vi "Main_EvaluateRotNoise.vi"() -> ()   [LabVIEW 2020]
panel:
  in  "Tab Control":T1(tab)
  in  "Num of Sim":i32=100
  out "XYグラフ":T2(graph)
  in  "Select Mol Posi":u16(ring)=4 items=["3-motors", "5-motors", "7-motors", "9-motors", "13-motors", "13-motors-sparse", "19-motors", ""]
  in  "SD":dbl=0.11000000000000001
  in  "Tau_On":i32=40
  in  "Tau_Off":i32=10
  in  "Sim time":i32=25000
  in  "Asymmetry (X, Y)":dbl[](array[numeric])=[0.12000000000000001, 0.58]
  out "Counter":i32
  in  "Torque":bool=TRUE
  in  "Torque (deg)":dbl=-4.0
  in  "停止":bool
  in  "Rot_Noise for Cargo":bool=TRUE
  in  "Width of Rot_Noise (deg)":dbl=8.0 format="%#_13g"
  in  "SaveData":bool
  out "Counter":i32
  in  "Ini_Posi (19 mol)":dbl[][](array[numeric])=[[0.0, 0.0], [12.0, 0.0], [-12.0, 0.0], [9.0, 3.0], [-9.0, 3.0], [9.0, -3.0], [-9.0, -3.0], [6.0, 0.0], [-6.0, 0.0], [0.0, 6.0], [0.0, -6.0], [6.0, 6.0], [6.0, -6.0], [-6.0, 6.0], [-6.0, -6.0], [3.0, 3.0], [3.0, -3.0], [-3.0, 3.0], [-3.0, -3.0]]
  in  "Ini_Posi (3 mol)":dbl[][](array[numeric])=[[0.0, 0.0], [6.0, 0.0], [-6.0, 0.0]]
  in  "Ini_Posi (5 mol)":dbl[][](array[numeric])=[[0.0, 0.0], [6.0, 0.0], [-6.0, 0.0], [0.0, 6.0], [0.0, -6.0]]
  in  "Ini_Posi (9 mol)":dbl[][](array[numeric])=[[0.0, 0.0], [6.0, 0.0], [-6.0, 0.0], [0.0, 6.0], [0.0, -6.0], [6.0, 6.0], [6.0, -6.0], [-6.0, 6.0], [-6.0, -6.0]]
  in  "Ini_Posi (13 mol)":dbl[][](array[numeric])=[[0.0, 0.0], [6.0, 0.0], [-6.0, 0.0], [0.0, 6.0], [0.0, -6.0], [6.0, 6.0], [6.0, -6.0], [-6.0, 6.0], [-6.0, -6.0], [3.0, 3.0], [3.0, -3.0], [-3.0, 3.0], [-3.0, -3.0]]
  in  "Ini_Posi (13 mol#2)":dbl[][](array[numeric])=[[0.0, 0.0], [17.0, 0.0], [-17.0, 0.0], [17.0, 9.0], [-17.0, 9.0], [17.0, -9.0], [-17.0, -9.0], [9.0, 0.0], [-9.0, 0.0], [9.0, 9.0], [9.0, -9.0], [-9.0, 9.0], [-9.0, -9.0]]
  in  "Ini_Posi (7 mol)":dbl[][](array[numeric])=[[0.0, 0.0], [5.0, 3.0], [-5.0, 3.0], [5.0, -3.0], [-5.0, -3.0], [0.0, 6.0], [0.0, -6.0]]
  out "Y":dbl[](graph)
  out "XY-trace":cluster{"Position":dbl[], "Position":dbl[]}[](graph)
  out "Angle":dbl[](graph)
  out "Num of On-Particles":dbl[](graph)
  out "Cross Corr":dbl[](graph)
  out "Corr_Coef_Pearson":T3
  out "Averaged CrossCorr":dbl[](graph)
  out "Graph_for_Coef":dbl[](graph)
  # "If you want to save data, press the button \nbefore you start simulations.\nSaved data contain time, Y-displacement, \nand angle."
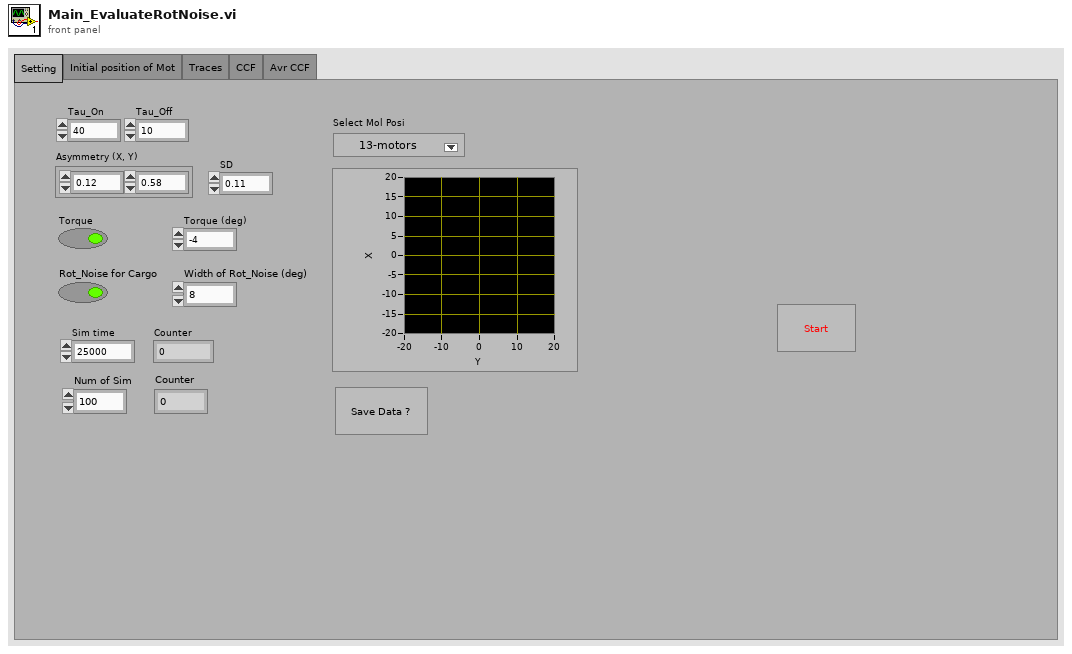
[diagram p1: front panel]
types:
  T1 = enum32{"Setting", "Initial position of Mot", "Traces", "CCF", "Avr CCF"}
  T2 = cluster{"Ini_Anchor_Posi (17 mol)":dbl[], "Ini_Anchor_Posi (17 mol)":dbl[]}
  T3 = cluster{"correlation coefficient r":dbl, "r^2":dbl}
  T4 = cluster{"Ini_Posi (19 mol) ":dbl[], "Ini_Posi (19 mol) ":dbl[]}
  T5 = cluster{"Center Position":dbl[], "Center Angle":dbl}
  T6 = cluster{"On/Off":bool, "Position":dbl[], "Dwell Count":i32}[]
  T7 = enum16{"open", "replace", "create", "open or create", "replace or create", "replace or create with confirmation"}
  T8 = cluster{"On/Off":bool, "Position":dbl[], "Next Dwell":i32}[]
  T9 = cluster{"On/Off":bool, "Position":dbl[], "Next Dwell":i32}
  T10 = cluster{"Center Position":dbl[], "Center Position":dbl[]}
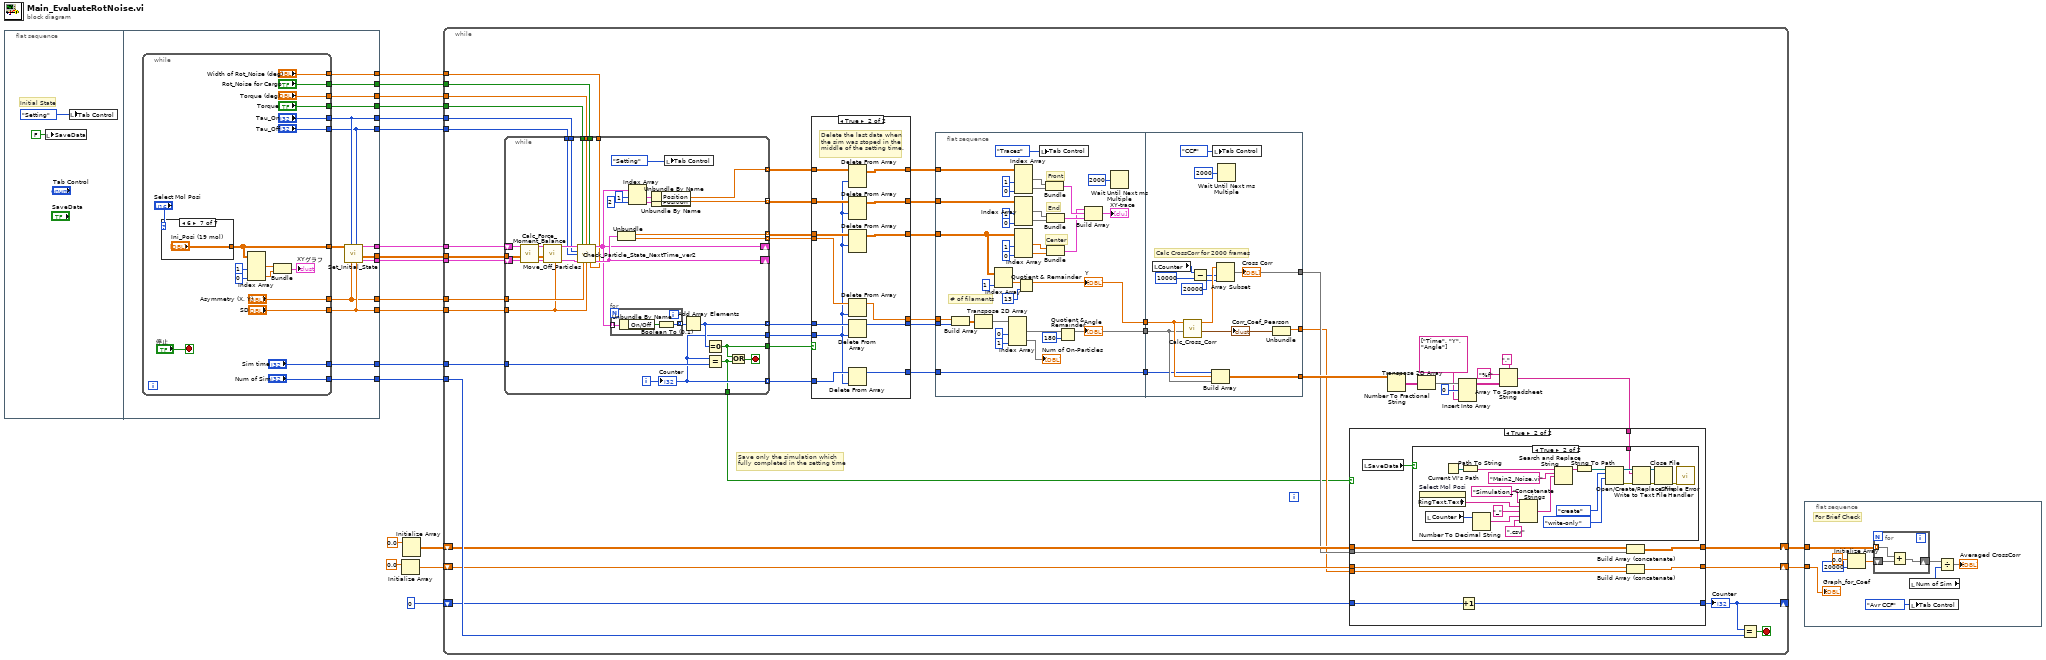
[diagram p0: block diagram]
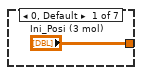
[diagram p5: hidden frame]
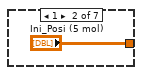
[diagram p6: hidden frame]
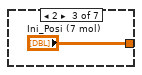
[diagram p7: hidden frame]
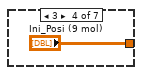
[diagram p8: hidden frame]
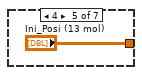
[diagram p9: hidden frame]
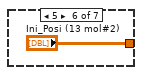
[diagram p10: hidden frame]
diagram:
  n1 = flat-sequence {
    tunnel: [w36] -> w20
    tunnel: [w35] -> w19
    tunnel: [w34] -> w18
    tunnel: [w31] -> w14
    tunnel: [w33] -> w17
    tunnel: [w32] -> w16
    tunnel: [w30] -> w15
    tunnel: [w29] -> w13
    tunnel: [w28] -> w12
    tunnel: [w26] -> w11
    tunnel: [w25] -> w10
    tunnel: [w24] -> w9
    tunnel: [w23] -> w8
    frame #0 {
      # "Initial State"
      n2 = local write "SaveData"(FALSE ("SaveData")) -> ()
      n3 = local write "Tab Control"(T1."Setting" ("Tab Control")) -> ()
    }
    frame #1 {
      n4 = while {
        tunnel: ["Tau_On"] -> w33
        tunnel: ["Tau_Off"] -> w32
        tunnel: ["SD"] -> w31
        tunnel: ["Asymmetry (X, Y)"] -> w30
        tunnel: ["Torque"] -> w29
        tunnel: ["Torque (deg)"] -> w28
        tunnel: [w48] -> w27
        tunnel: ["Rot_Noise for Cargo"] -> w26
        tunnel: ["Width of Rot_Noise (deg)"] -> w25
        tunnel: ["Sim time"] -> w24
        tunnel: ["Num of Sim"] -> w23
        stop <- "停止" stop-if-true
        n5 = case shown="6" "Select Mol Posi" {
          tunnel: ["Ini_Posi (3 mol)" "Ini_Posi (5 mol)" "Ini_Posi (7 mol)" "Ini_Posi (9 mol)" "Ini_Posi (13 mol)" "Ini_Posi (13 mol#2)" "Ini_Posi (19 mol)"] -> w48
          frame 0, Default {
          }
          frame 1 {
          }
          frame 2 {
          }
          frame 3 {
          }
          frame 4 {
          }
          frame 5 {
          }
          frame 6 {
          }
        }
        n6 = Index Array(array=w48, index (col) #1=1 ("無効な指標 (列)"), index (col) #2=0 ("指標 (列)")) -> (element #1=w43:dbl[], element #2=w42:dbl[])  [unwired: 2 in]
        n7 = Bundle("Ini_Posi (19 mol)"=w43, "Ini_Posi (19 mol)"=w42) -> (→"XYグラフ":T4)  [unwired: 1 in]
      }
      n8 = call "Set_Initial_State.vi"("SD"=w31, "Tau_Off"=w32, "Asymmetry (X, Y)"=w30, "Tau_On"=w33, "Ini_Anchor_Posi"=w27) -> ("Center State at T"=w34:T5, "Ini_Anchor_Posi"=w35:dbl[][], "On_Particle State"=w36:T6)  [unwired: 4 in]
    }
  }
  n9 = Initialize Array(0.0 ("要素")) -> (w6:dbl[])  [unwired: 1 in]
  n10 = Initialize Array(0.0 ("要素")) -> (w4:dbl[][])  [unwired: 2 in]
  n11 = while {
    tunnel: w20 -> [w110]
    tunnel: w19 -> [w109]
    tunnel: w18 -> [w108]
    tunnel: w17 -> [w107]
    tunnel: w16 -> [w106]
    tunnel: w15 -> [w105]
    tunnel: w14 -> [w104]
    tunnel: w13 -> [w103]
    tunnel: w12 -> [w102]
    tunnel: w11 -> [w96]
    tunnel: w10 -> [w95]
    tunnel: w9 -> [w94]
    tunnel: w8 -> [w92]
    shift-right: [w67] -> w2
    shift-left: w6 -> [w68]
    shift-right: [w70] -> w3
    shift-left: w4 -> [w69]
    shift-right: [w63] -> _
    shift-left: 0 -> [w64]
    stop <- w93 stop-if-true
    # "Save only the simulation which \nfully completed in the setting time"
    n12 = while {
      tunnel: w109 -> [w195]
      shift-right: [w186] -> _
      shift-left: w108 -> [w193]
      shift-right: [w179] -> _
      shift-left: w110 -> [w194]
      tunnel: w107 -> [w185]
      tunnel: w106 -> [w184]
      tunnel: w105 -> [w181]
      tunnel: w104 -> [w180]
      tunnel: w103 -> [w182]
      tunnel: w102 -> [w183]
      tunnel: w94 -> [w166]
      tunnel: [w174] -> w89
      tunnel: [w165] -> w88
      tunnel: w96 -> [w173]
      tunnel: w95 -> [w172]
      tunnel: [w171] -> w87 mode=indexing
      tunnel: [w170] -> w86 mode=indexing
      tunnel: [w169] -> w85 mode=indexing
      tunnel: [w168] -> w84 mode=indexing
      tunnel: [w167] -> w83 mode=indexing
      tunnel: [w165] -> w82 mode=indexing
      tunnel: [w164] -> w62
      i -> [w165]
      stop <- w175 stop-if-true
      n13 = call "Calc_Force_Moment_Balance.vi"("Center State at T"=w193, "Ini_Anchor_Posi"=w195, "On_Particle State"=w194) -> ("New Center State at T"=w188:T5, "Ini_Anchor_Posi"=w189:dbl[][], "On_Particle State"=w196:T6)  [unwired: 6 in]
      n14 = call "Move_Off_Particles.vi"("SD"=w180, "Center State at T"=w188, "Ini_Anchor_Posi"=w189, "Particle Posi at T"=w196) -> ("Center State at T"=w187:T5, "New Particle Posi at T"=w190:T8)  [unwired: 6 in]
      n15 = call "Check_Particle_State_NextTime_ver2.vi"("Particle State at T"=w190, "Torque?"=w182, "Torque"=w183, "Rot diffusion\nfor Cargo?"=w173, "Tau_On"=w185, "Tau_Off"=w184, "Center State at T"=w187, "Asymmetry (X, Y)"=w181, "SD"=w180, "Rot diffusion\nfor Cargo"=w172) -> ("Particle State at T+1"=w179:T8, "New Center State at T"=w186:T5)  [unwired: 4 in]
      n16 = for {
        tunnel: w179 -> [w199] mode=indexing
        tunnel: [w197] -> w178 mode=indexing
        n17 = Unbundle By Name(w199) -> ("On/Off"=w198:bool)
        n18 = Boolean To (0,1)(Boolean=w198) -> (0, 1=w197:i16)
      }
      n19 = Unbundle(w186) -> ("Center Position"=w169:dbl[], "Center Angle"=w168:dbl)
      n20 = Index Array(array=w179, index #1=1 ("index"), index #2=2 ("index")) -> (element #1=w192:T9, element #2=w191:T9)
      n21 = Unbundle By Name(w192) -> ("Position"=w171:dbl[])
      n22 = Unbundle By Name(w191) -> ("Position"=w170:dbl[])
      n23 = local write "Tab Control"(T1."Setting" ("Tab Control")) -> ()
      n24 = Add Array Elements(numeric array=w178) -> (sum=w167:i16)
      n25 = Equal To 0?(x=w167) -> (x = 0?=w174:bool)
      n26 = Equal?(x=w165, y=w166) -> (x = y?=w164:bool)
      n27 = Or(x=w174, y=w164) -> (x .or. y?=w175:bool)
      "Counter" <- w165
    }
    n28 = case shown="TRUE" w89 {
      tunnel: w87 -> [w149 w162]
      tunnel: w86 -> [w148 w161]
      tunnel: w88 -> [_ w151]
      tunnel: w85 -> [w147 w160]
      tunnel: w84 -> [w146 w159]
      tunnel: w83 -> [w145 w158]
      tunnel: [w145 w157] -> w101
      tunnel: [w146 w156] -> w100
      tunnel: [w147 w155] -> w99
      tunnel: [w148 w154] -> w98
      tunnel: [w149 w153] -> w97
      tunnel: w82 -> [w144 w152]
      tunnel: [w144 w150] -> w81
      frame False {
      }
      frame True {
        # "Delete the last data when \nthe sim was stoped in the\nmiddle of the setting time."
        n29 = Delete From Array(array=w162, index (row)=w151) -> (array with subset deleted=w153:dbl[][])  [unwired: 2 in, 1 out]
        n30 = Delete From Array(array=w161, index (row)=w151) -> (array with subset deleted=w154:dbl[][])  [unwired: 2 in, 1 out]
        n31 = Delete From Array(array=w160, index (row)=w151) -> (array with subset deleted=w155:dbl[][])  [unwired: 2 in, 1 out]
        n32 = Delete From Array(array=w159, index=w151) -> (array with subset deleted=w156:dbl[])  [unwired: 1 in, 1 out]
        n33 = Delete From Array(array=w158, index=w151) -> (array with subset deleted=w157:i16[])  [unwired: 1 in, 1 out]
        n34 = Delete From Array(array=w152, index=w151) -> (array with subset deleted=w150:i32[])  [unwired: 1 in, 1 out]
      }
    }
    n35 = flat-sequence {
      tunnel: w101 -> [w235]
      tunnel: w100 -> [w234]
      tunnel: w99 -> [w206]
      tunnel: w98 -> [w207]
      tunnel: w97 -> [w208]
      tunnel: [w204] -> w91
      tunnel: [w203] -> w90
      tunnel: w81 -> [w202]
      tunnel: [w202] -> w80
      tunnel: [w244] -> w66
      tunnel: w91 -> [w239]
      tunnel: w90 -> [w240]
      tunnel: [w241] -> w65
      tunnel: [w238] -> w79
      tunnel: w80 -> [w237]
      frame #0 {
        # "End"
        # "Front"
        # "Center"
        # "# of filaments"
        n36 = Build Array(w234, w235) -> (w233:dbl[][])
        n37 = Transpose 2D Array(2D array=w233) -> (transposed array=w205:dbl[][])
        n38 = Index Array(array=w206, index (col)=1 ("disabled index (col)")) -> (element=w226:dbl[])  [unwired: 1 in]
        n39 = Index Array(array=w205, index (col) #1=0 ("disabled index (col)"), index (col) #2=1 ("index (col)")) -> (element #1=w228:dbl[], element #2=→"Num of On-Particles":dbl[])  [unwired: 2 in]
        n40 = Index Array(array=w208, index (col) #1=1 ("disabled index (col)"), index (col) #2=0 ("index (col)")) -> (element #1=w212:dbl[], element #2=w221:dbl[])  [unwired: 2 in]
        n41 = Index Array(array=w207, index (col) #1=1 ("disabled index (col)"), index (col) #2=0 ("index (col)")) -> (element #1=w213:dbl[], element #2=w220:dbl[])  [unwired: 2 in]
        n42 = Index Array(array=w206, index (col) #1=1 ("disabled index (col)"), index (col) #2=0 ("index (col)")) -> (element #1=w211:dbl[], element #2=w215:dbl[])  [unwired: 2 in]
        n43 = Quotient & Remainder(x=w226, y=13) -> (x-y*floor(x/y)=w203:dbl[])  [unwired: 1 out]
        "Y" <- w203
        n44 = local write "Tab Control"(T1."Traces" ("Tab Control")) -> ()
        n45 = Bundle("Position"=w212, "Position"=w221) -> (w219:cluster{"Position":dbl[], "Position":dbl[]})  [unwired: 1 in]
        n46 = Bundle("Position"=w213, "Position"=w220) -> (w218:cluster{"Position":dbl[], "Position":dbl[]})  [unwired: 1 in]
        n47 = Bundle("Center Position"=w211, "Center Position"=w215) -> (w214:T10)  [unwired: 1 in]
        n48 = Quotient & Remainder(x=w228, y=180) -> (x-y*floor(x/y)=w204:dbl[])  [unwired: 1 out]
        "Angle" <- w204
        n49 = Build Array(w214, w219, w218) -> (→"XY-trace":cluster{"Position":dbl[], "Position":dbl[]}[])
        n50 = Wait Until Next ms Multiple(millisecond multiple=u32 2000 ("ミリ秒倍数")) -> ()  [unwired: 1 out]
      }
      frame #1 {
        # "Calc CrossCorr for 2000 frames"
        n51 = local read "Counter"() -> (w243:i32)
        n52 = call "Calc_Cross_Corr.vi"("Y"=w239, "X"=w240) -> ("Corr_Coef_Pearson"=w242:T3, "Cross"=w248:dbl[])  [unwired: 7 in, 1 out]
        "Corr_Coef_Pearson" <- w242
        n53 = Subtract(x=w243, y=10000) -> (x-y=w245:i32)
        n54 = Build Array(w237, w240, w239) -> (w238:dbl[][])
        n55 = local write "Tab Control"(T1."CCF" ("Tab Control")) -> ()
        n56 = Array Subset(array=w248, index=w245, length=20000 ("長さ")) -> (w244:dbl[])
        "Cross Corr" <- w244
        n57 = Wait Until Next ms Multiple(millisecond multiple=u32 2000 ("ミリ秒倍数")) -> ()  [unwired: 1 out]
        n58 = Unbundle(w242) -> ("correlation coefficient r"=w241:dbl)  [unwired: 1 out]
      }
    }
    n59 = Number To Fractional String(number=w79) -> (F-format string=w75:string[][])  [unwired: 3 in]
    n60 = Transpose 2D Array(2D array=w75) -> (transposed array=w78:string[][])
    n61 = Insert Into Array(array=w78, index (row)=0 ("指標 (行)"), new element=string[] ["Time", "Y", "Angle"]) -> (w73:string[][])  [unwired: 1 in]
    n62 = Array To Spreadsheet String(delimiter (Tab)=",", array=w73, 3:"%f" ("format string")) -> (spreadsheet string=w72:string)
    n63 = case shown="TRUE" w62 {
      tunnel: w72 -> [_ w123]
      tunnel: [w113 w121] -> w70
      tunnel: w69 -> [w113 w122]
      tunnel: [w112 w118] -> w67
      tunnel: w68 -> [w112 w119]
      tunnel: w66 -> [_ w120]
      tunnel: w65 -> [_ w117]
      tunnel: [w111 w116] -> w63
      tunnel: w64 -> [w111 w115]
      frame False {
      }
      frame True {
        n64 = local read "SaveData"() -> (w114:bool)
        n65 = case shown="TRUE" w114 {
          tunnel: w123 -> [_ w128]
          frame False {
          }
          frame True {
            n66 = property on="Select Mol Posi" class="Ring (指定)"() -> ("RingText.Text"=w129:string)  [unwired: 2 in, 2 out]
            n67 = local read "Counter"() -> (w127:i32)
            n68 = Current VI's Path() -> (path=w135:path)
            n69 = Path To String(path=w135) -> (string=w134:string)
            n70 = Number To Decimal String(number=w127) -> (decimal integer string=w125:string)  [unwired: 1 in]
            n71 = Concatenate Strings("Simulation_" ("文字列"), w129, "_" ("文字列"), w125, ".csv" ("string")) -> (w132:string)
            n72 = Search and Replace String(input string=w134, search string="Main2_Noise.vi", replace string=w132) -> (result string=w131:string)  [unwired: 5 in, 3 out]
            n73 = String To Path(string=w131) -> (path=w136:path)
            n74 = Open/Create/Replace File(file path (use dialog)=w136, operation (0:open)=T7."create", access (0:read/write)=enum16{"read/write", "read-only", "write-only"}."write-only") -> (refnum out=w139:refnum<file>, error out=w140:errorcluster)  [unwired: 1 in, 3 out]
            n75 = Write to Text File(file (use dialog)=w139, text=w128, error in=w140) -> (refnum out=w142:refnum<file>, error out=w143:errorcluster)  [unwired: 1 in, 1 out]
            n76 = Close File(refnum=w142, error in=w143) -> (error out=w141:errorcluster)  [unwired: 1 out]
            n77 = call <vilib>:"Simple Error Handler.vi"("error in (no error)"=w141) -> ()  [unwired: 1 in, 8 out]
          }
        }
        n78 = Increment(x=w115) -> (x+1=w116:i32)
        n79 = Build Array (concatenate)(w122, w120) -> (w121:dbl[][])
        n80 = Build Array (concatenate)(w119, w117) -> (w118:dbl[])
      }
    }
    "Counter" <- w63
    n81 = Equal?(x=w63, y=w92) -> (x = y?=w93:bool)
  }
  n82 = flat-sequence {
    tunnel: w3 -> [w258]
    tunnel: w2 -> [w251]
    frame #0 {
      # "For Brief Check"
      n83 = Initialize Array(0.0 ("要素"), 20000 ("次元サイズ")) -> (w256:dbl[])
      n84 = for {
        tunnel: w258 -> [w261] mode=indexing
        shift-right: [w259] -> w254
        shift-left: w256 -> [w260]
        n85 = Add(x=w261, y=w260) -> (x+y=w259:dbl[])
      }
      n86 = local read "Num of Sim"() -> (w253:i32)
      n87 = local write "Tab Control"(T1."Avr CCF" ("Tab Control")) -> ()
      n88 = Divide(x=w254, y=w253) -> (x/y=→"Averaged CrossCorr":dbl[])
      "Graph_for_Coef" <- w251
    }
  }
